vi "Manual.vi"(8 "error in (no error)":errorcluster, 10 "Mirrors":T1, 11 "Flip Mirror Containter in":refnum<class "Flip Mirror Containter.lvclass">) -> (0 "error out":errorcluster, 3 "Flip Mirror Containter out":refnum<class "Flip Mirror Containter.lvclass">)   [LabVIEW 2016, in "Flip Mirror Containter.lvclass"]
uses:
  Flip Mirror Containter.lvclass
  Controls/Flip Mirrors.ctl
  Controls/Mirror Data.ctl
  Flip Mirror Containter.lvclass/Flip Mirror Containter.ctl
  SolarMir.lvclass
  ThArMir.lvclass
  ExtFlatMir.lvclass
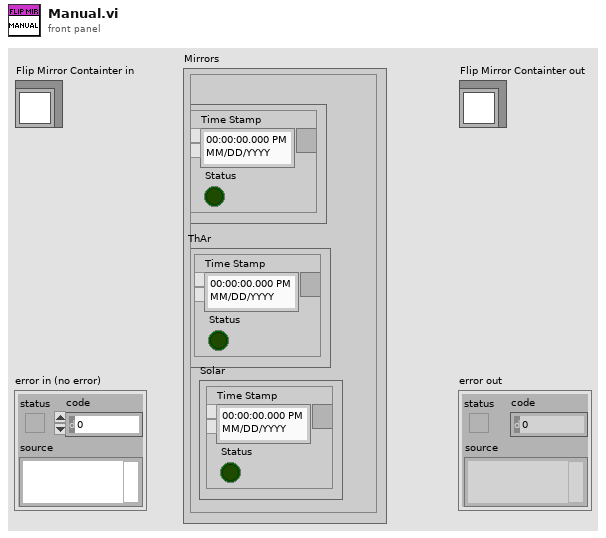
[diagram p1: front panel]
types:
  T1 = typedef "Flip Mirrors.ctl" = cluster{"ExtFlat":T2, "ThAr":T2, "Solar":T2}
  T2 = typedef "Mirror Data.ctl" = cluster{"Status":bool, "Time Stamp":timestamp}
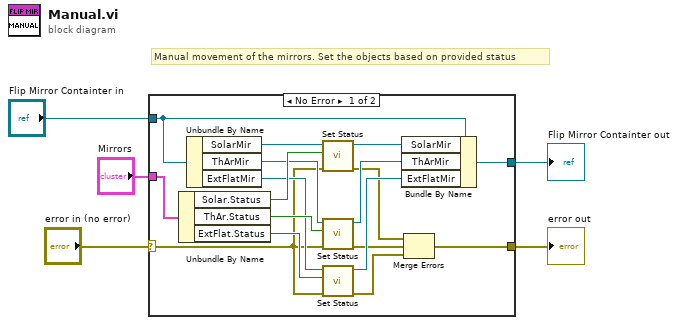
[diagram p0: block diagram]
diagram:
  # "Manual movement of the mirrors. Set the objects based on provided status"
  n1 = case shown="No Error" "error in (no error)" {
    selector: "error in (no error)" -> [w10 w24]
    tunnel: [w9 w24] -> w4
    tunnel: [w20 w23] -> w2
    tunnel: "Flip Mirror Containter in" -> [w21 w23]
    tunnel: "Mirrors" -> [w22 _]
    frame No Error {
      n2 = Unbundle By Name(w22) -> ("Solar.Status"=w18:bool, "ThAr.Status"=w16:bool, "ExtFlat.Status"=w14:bool)
      n3 = Unbundle By Name(w21) -> ("SolarMir"=w19:refnum<class "SolarMir.lvclass">, "ThArMir"=w17:refnum<class "ThArMir.lvclass">, "ExtFlatMir"=w15:refnum<class "ExtFlatMir.lvclass">)
      n4 = call-dynamic "Set Status.vi"("error in (no error)"=w10, "Status"=w18, "FlipMir in"=w19) -> ("error out"=w8:errorcluster, "FlipMir out"=w13:refnum<class "SolarMir.lvclass">)  [unwired: 7 in]
      n5 = call-dynamic "Set Status.vi"("error in (no error)"=w10, "Status"=w16, "FlipMir in"=w17) -> ("error out"=w7:errorcluster, "FlipMir out"=w12:refnum<class "ThArMir.lvclass">)  [unwired: 7 in]
      n6 = call-dynamic "Set Status.vi"("error in (no error)"=w10, "Status"=w14, "FlipMir in"=w15) -> ("error out"=w6:errorcluster, "FlipMir out"=w11:refnum<class "ExtFlatMir.lvclass">)  [unwired: 7 in]
      n7 = Bundle By Name(cluster=w21, "SolarMir"=w13, "ThArMir"=w12, "ExtFlatMir"=w11) -> (w20:refnum<class "Flip Mirror Containter.lvclass">)
      n8 = Merge Errors(w8, w7, w6) -> (w9:errorcluster)
    }
    frame Error {
    }
  }
  "error out" <- w4
  "Flip Mirror Containter out" <- w2
